vi "Add New product.vi"(8 "error in (no error)":errorcluster, 11 "Module Number  2":dbl=1.0) -> (0 "error out":errorcluster, 2 "Sucess ?":bool, 3 "subarray":string[](array[string]))   [LabVIEW 2015, in "Copy of Untitled Library 1.lvlib"]
uses:
  Copy of Untitled Library 1.lvlib
  Controls/Caller Queue Control .ctl
  Controls/Control 1.ctl
  Controls/Enum Constant.ctl
  <userlib>/origin_lib_main/db_interface/DB Operations Enum.ctl
  <userlib>/origin_lib_main/ui_msg_lib/CTRL/Display MSG Types.ctl
  <userlib>/origin_lib_main/ui_msg_lib/MSG Library.lvlib
  <userlib>/origin_lib_main/db_interface/DB Interface.lvlib
panel:
  in  "Cluster":T1
  in  "error in (no error) 5":errorcluster
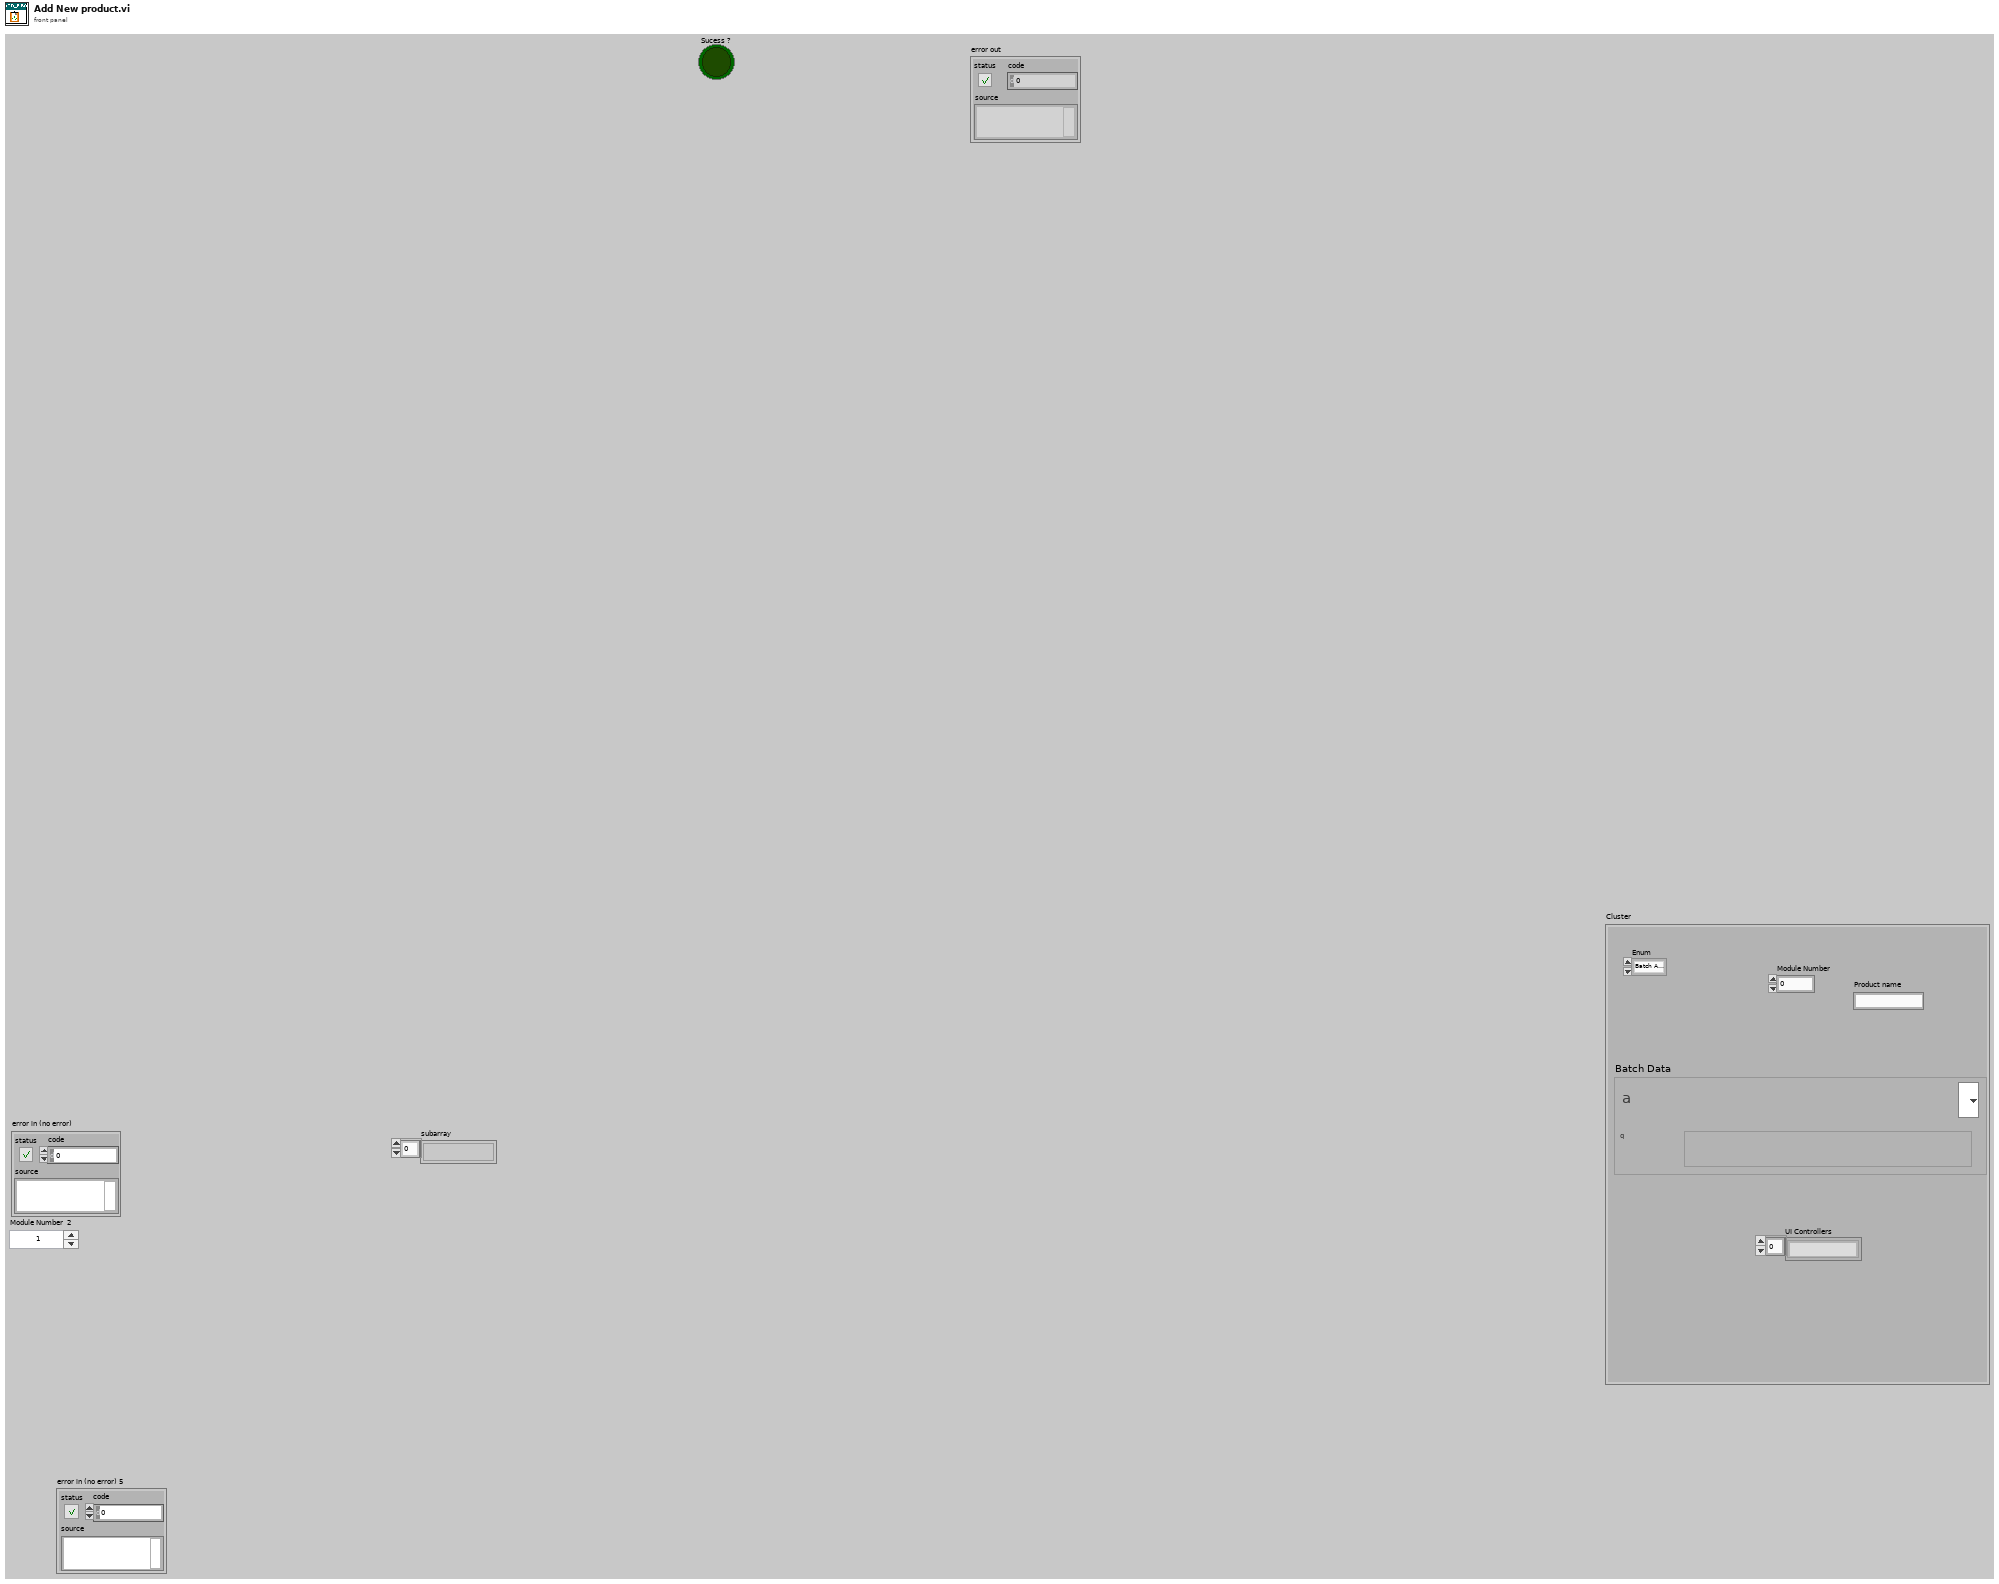
[diagram p1: front panel]
types:
  T1 = typedef "Caller Queue Control .ctl" = cluster{"Enum":enum16{"Batch Added", "Batch Deleted", "Batch Opened", "Batch Closed", "Batch Edited", "new Product Added", "Product deleted "}, "Batch Data 3":T2, "UI Controllers":string[], "Product name":string, "Module Number":dbl}
  T2 = typedef "Copy of Untitled Library 1.lvlib/Control 1.ctl" = cluster{"DATA":string, "DATA 2":string, "DATA 3":string, "DATA 4":string, "DATA 5":string, "DATA 6":string, "DATA 7":string, "DATA 8":string, "DATA 9":string, "DATA 10":string, "Product":string}
  T3 = typedef "DB Interface.lvlib/DB Operations Enum.ctl" = enum16{"Select", "Update", "Insert", "Delete", "Fetch SQL Query", "Execute SQL Query", "Drop Table", "List Tables"}
  T4 = typedef "Enum Constant.ctl" = enum16{"Init", "Read", "Write"}
  T5 = typedef "MSG Library.lvlib/Display MSG Types.ctl" = enum16{"Display MSG 1", "Display MSG 2", "Display MSG Load", "End MSG Load ", "Display 2 STR MSG"}
  T6 = typedef "FGV Data.ctl" = T7[]
  T7 = typedef "FGV Cluster Data.ctl" = cluster{"Manual/Automatic":bool, "UI Controllers ":string[], "UI Primery Key ":dbl[], "Caller Queue & MSG":T8, "Module ID":dbl, "DB Reference In":T9, "Products Columns":string[], "Cluster":cluster{"Delete Product":enum8{"Enabled", "Disabled", "Disabled and Grayed Out"}, "Add Product ":enum8{"Enabled", "Disabled", "Disabled and Grayed Out"}, "EDIT BATCH":enum8{"Enabled", "Disabled", "Disabled and Grayed Out"}, "Open Batch ":enum8{"Enabled", "Disabled", "Disabled and Grayed Out"}, "Close Batch":enum8{"Enabled", "Disabled", "Disabled and Grayed Out"}, "Delete Batch":enum8{"Enabled", "Disabled", "Disabled and Grayed Out"}, "Add Batch ":enum8{"Enabled", "Disabled", "Disabled and Grayed Out"}}}
  T8 = typedef "Queue and Caller MSG.ctl" = cluster{"Caller Queue":refnum<queue>, "Caller MSG":string}
  T9 = typedef "NI_Database_API.lvlib/Conn ObjectReference.ctl" = refnum<k1>
  T10 = enum16{"Batch Added", "Batch Deleted", "Batch Opened", "Batch Closed", "Batch Edited", "new Product Added", "Product deleted "}
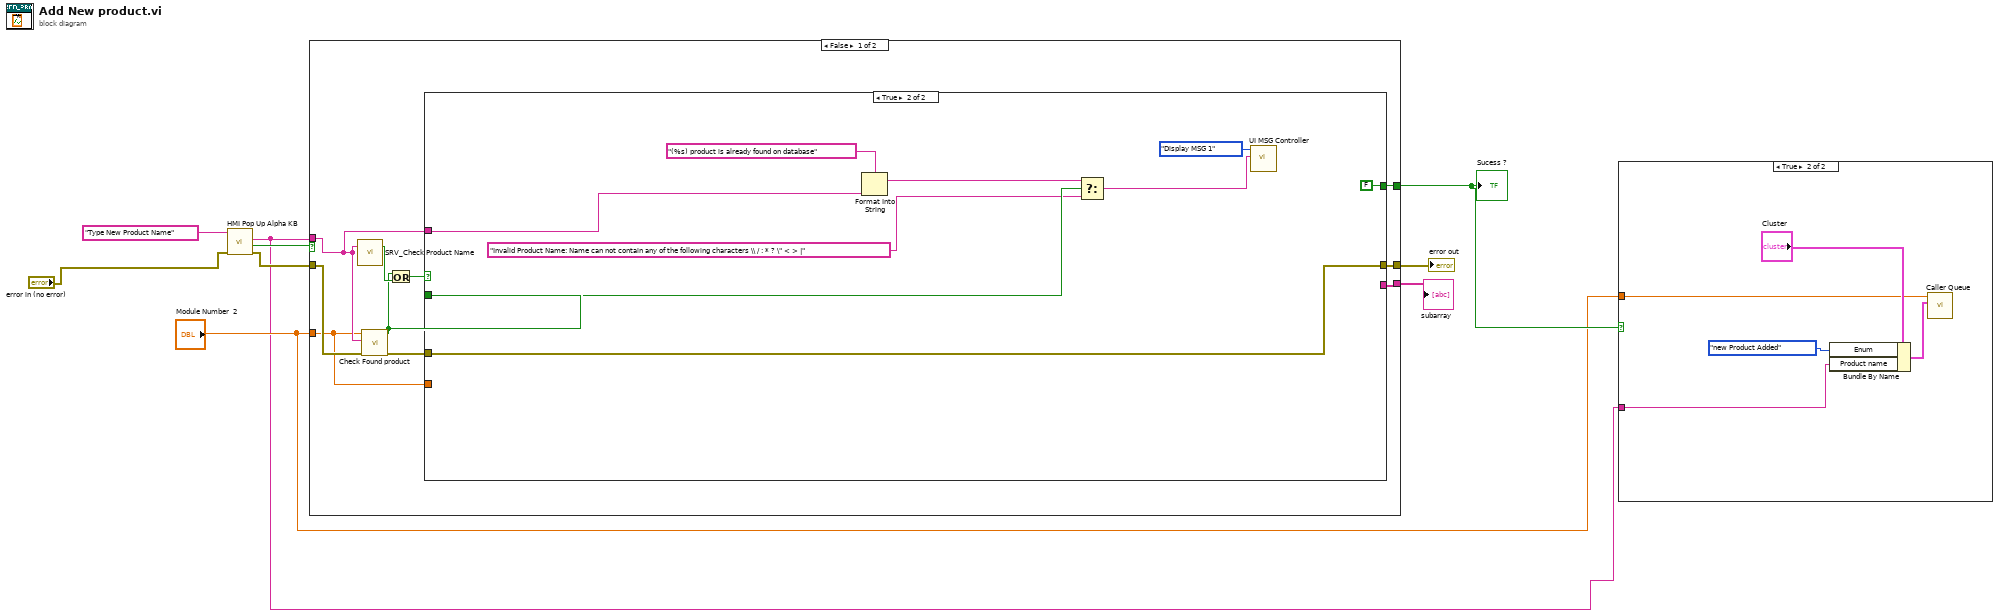
[diagram p0: block diagram]
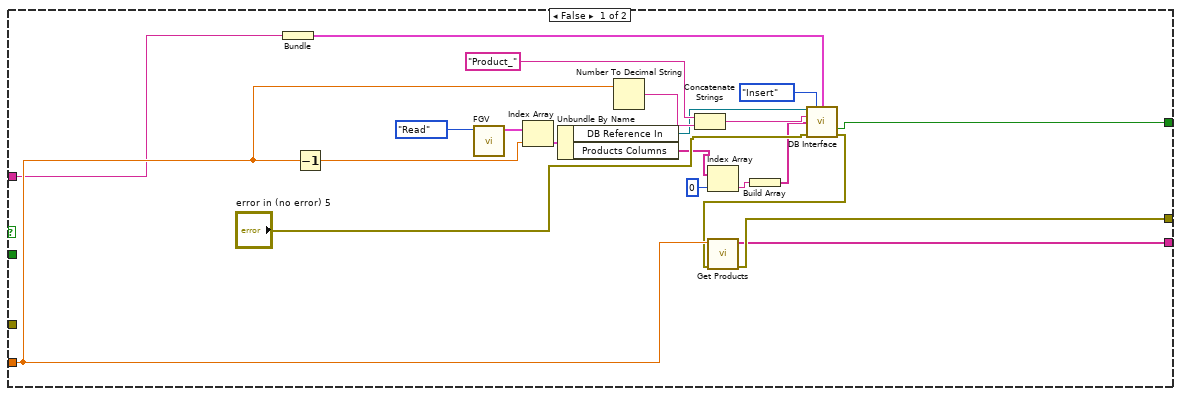
[diagram p3: hidden frame]
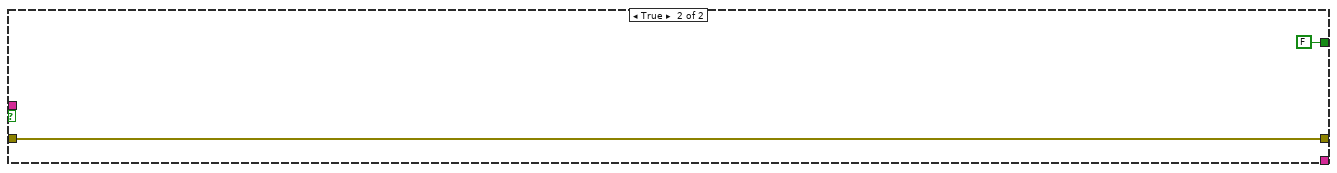
[diagram p4: hidden frame]
diagram:
  n1 = call "HMI Pop Up Alpha KB.vi"("error in (no error)"="error in (no error)", "Message In"="Type New Product Name") -> ("error out"=w7:errorcluster, "Canceled"=w8:bool, "String Out"=w1:string)  [unwired: 7 in]
  n2 = case shown="False" w8 {
    tunnel: w1 -> [w16 _]
    tunnel: w7 -> [w14 w51]
    tunnel: [w17 w51] -> w4
    tunnel: "Module Number  2" -> [w12 _]
    tunnel: [w11 _] -> w5
    tunnel: [w10 FALSE ("Sucess ?")] -> w3
    frame False {
      n3 = call "SRV_Check Product Name.vi"("String"=w16) -> ("Not Valid"=w18:bool)  [unwired: 2 in]
      n4 = call "Check Found product.vi"("error in (no error) 5"=w14, "Product Name"=w16, "Module Number  2"=w12) -> ("error out 2"=w13:errorcluster, "Found 2"=w15:bool)  [unwired: 7 in]
      n5 = Or(x=w15, y=w18) -> (x .or. y?=w19:bool)
      n6 = case shown="True" w19 {
        tunnel: w16 -> [w22 w49]
        tunnel: [w40 w46] -> w17
        tunnel: w15 -> [_ w47]
        tunnel: w13 -> [_ w46]
        tunnel: w12 -> [w28 _]
        tunnel: [w39 _] -> w11
        tunnel: [w20 FALSE ("Sucess ?")] -> w10
        frame False {
          n7 = Bundle("String Out"=w22) -> (w21:cluster{"String Out":string})  [unwired: 1 in]
          n8 = Decrement(x=w28) -> (x-1=w31:dbl)
          n9 = call "FGV.vi"("Enum"=Enum_Constant."Read") -> ("Read Data"=w33:T6)  [unwired: 9 in, 1 out]
          n10 = Index Array(array=w33, index=w31) -> (element=w32:T7)
          n11 = Unbundle By Name(w32) -> ("DB Reference In"=w30:T9, "Products Columns"=w27:string[])
          n12 = Number To Decimal String(number=w28) -> (decimal integer string=w35:string)  [unwired: 1 in]
          n13 = Concatenate Strings("Product_" ("string"), w35) -> (w34:string)
          n14 = Index Array(array=w27, index=0) -> (element=w25:string)
          n15 = Build Array(w25) -> (w24:string[])
          n16 = call <userlib>:"DB Interface.vi"("DB Ref In"=w30, "Operation"=DB_Operations_Enum."Insert", "data"=w21, "DB Table"=w34, "DB columns"=w24, "error in (no error)"="error in (no error) 5") -> ("Sucess ?"=w20:bool, "error out"=w23:errorcluster)  [unwired: 6 in, 2 out]
          n17 = call "Get Products.vi"("error in (no error) 5"=w23, "Module Number  2"=w28) -> ("error out 2"=w40:errorcluster, "subarray"=w39:string[])  [unwired: 8 in]
        }
        frame True {
          n18 = Format Into String(format string="(%s) product is already found on database", w49) -> (resulting string=w48:string)  [unwired: 2 in, 1 out]
          n19 = Select(t=w48, s=w47, f="Invalid Product Name: Name can not contain any of the following characters \\ / : * ? \" < > |" ("format string")) -> (s? t:f=w44:string)
          n20 = call <userlib>:"UI MSG Controller.vi"("MSG"=w44, "Display MSG Type"=Display_MSG_Types."Display MSG 1") -> ()  [unwired: 6 in, 4 out]
        }
      }
    }
    frame True {
    }
  }
  "error out" <- w4
  "subarray" <- w5
  "Sucess ?" <- w3
  n21 = case shown="True" w3 {
    tunnel: "Module Number  2" -> [_ w54]
    tunnel: w1 -> [_ w53]
    frame False {
    }
    frame True {
      n22 = Bundle By Name(cluster="Cluster", "Enum"=T10."new Product Added", "Product name"=w53) -> (w52:T1)
      n23 = call "Caller Queue .vi"("Cluster"=w52, "Module Number  3"=w54) -> ()  [unwired: 9 in, 1 out]
    }
  }
